vi "0716206_calculator_without_formula.vi"() -> ()   [LabVIEW 2021]
uses:
  <vilib>/Utility/miscctls.llb/LVDateTimeRec.ctl
panel:
  out "date time rec":T1
  out "stack":dbl[](array[numeric])
  out "is_neg":bool=TRUE
  out "Array operator":string[](array[string])
  out "buffer":string
  out "Array number":dbl[](array[numeric])
  out "Power":bool
  out "Storage2 ans":dbl format="%#_13g"
  out "Storage1 ans":dbl format="%#_13g"
  out "B":bool=TRUE
  out "Storage2":string
  out "Storage1":string
  out "Error":string
  out "Ans":dbl format="%#_13g"
  out "System Time":string
  out "Execution Time (s)":dbl caption="Elapsed Time (s)"
  out "String":string
  in  "Cluster":T2
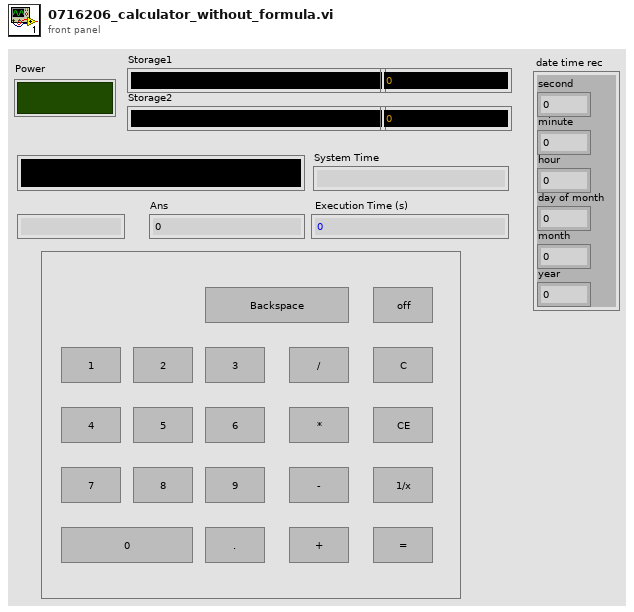
[diagram p1: front panel]
types:
  T1 = typedef "LVDateTimeRec.ctl" = cluster{"fractional second":dbl, "second":i32, "minute":i32, "hour":i32, "day of month":i32, "month":i32, "year":i32, "day of week":i32, "day of year":i32, "DST":i32}
  T2 = cluster{bool, bool, bool, bool, bool, bool, bool, bool, bool, bool, bool, bool, bool, bool, bool, bool, bool, bool, bool, bool, bool, bool, bool, bool}
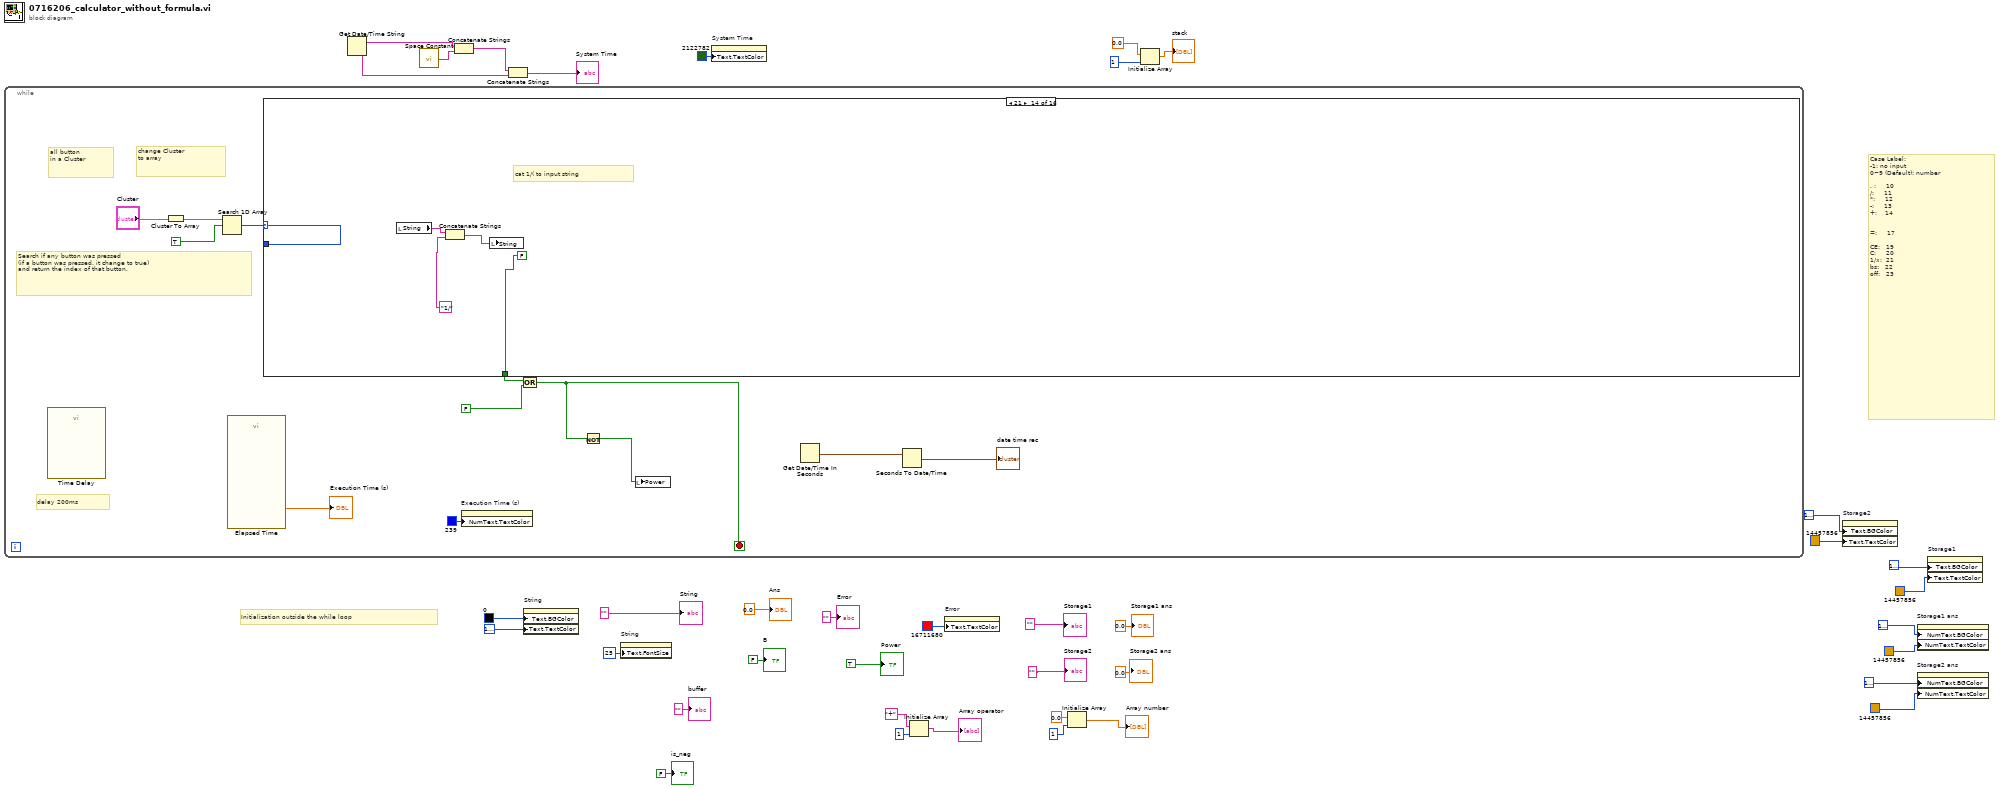
[diagram p0: block diagram]
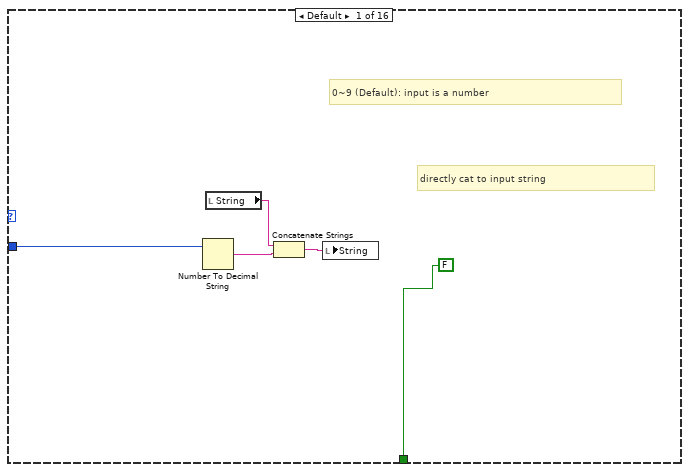
[diagram p2: hidden frame]
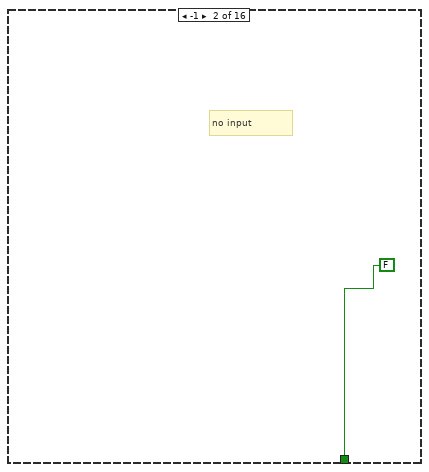
[diagram p3: hidden frame]
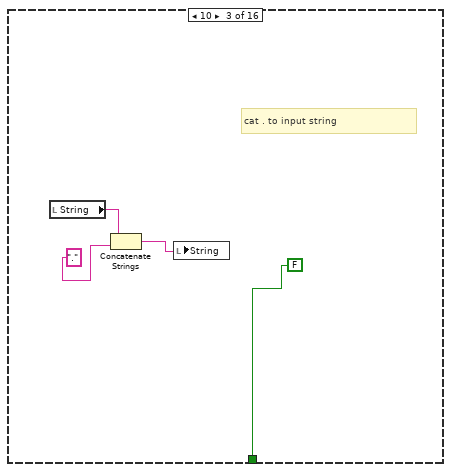
[diagram p4: hidden frame]
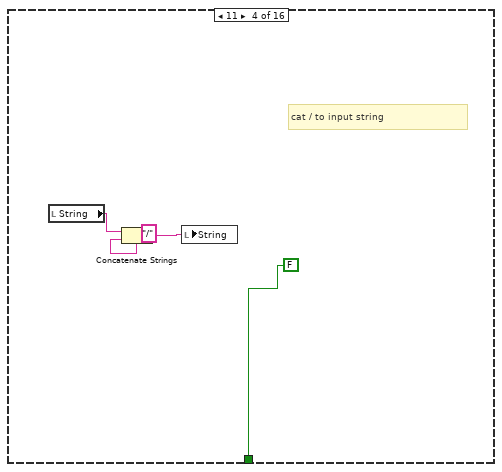
[diagram p5: hidden frame]
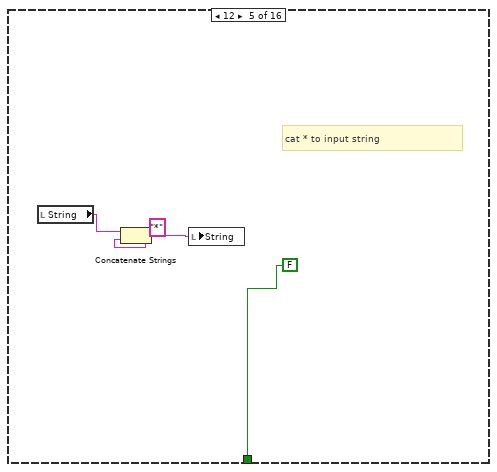
[diagram p6: hidden frame]
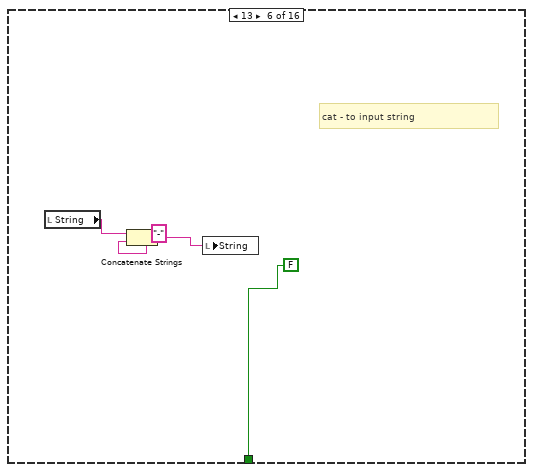
[diagram p7: hidden frame]
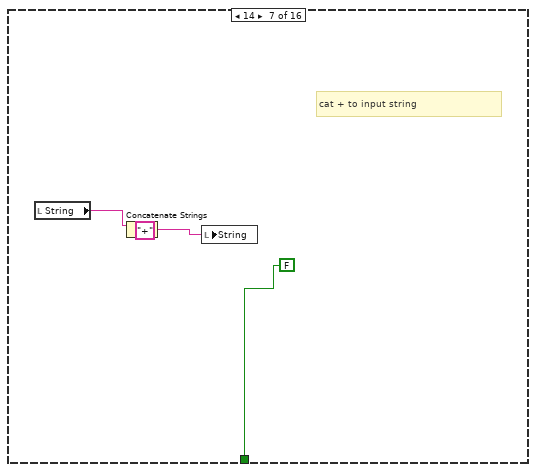
[diagram p8: hidden frame]
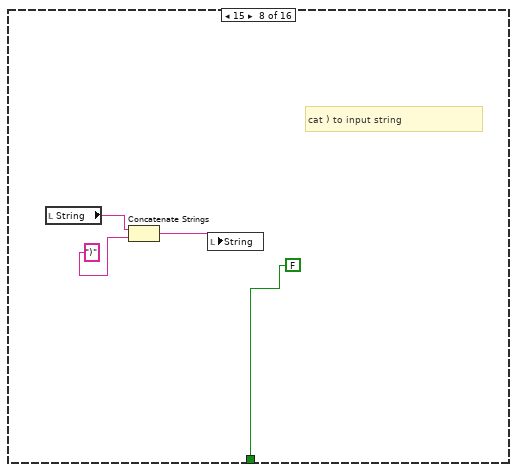
[diagram p9: hidden frame]
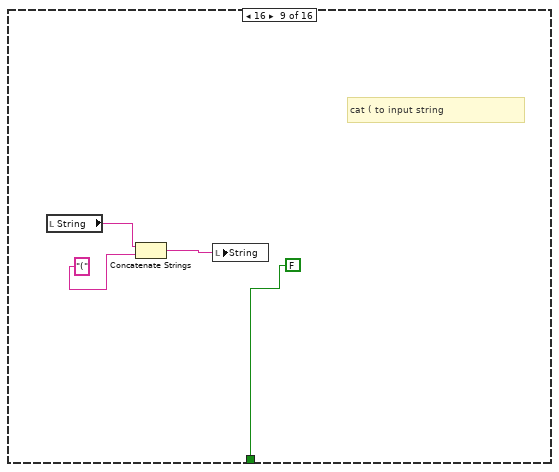
[diagram p10: hidden frame]
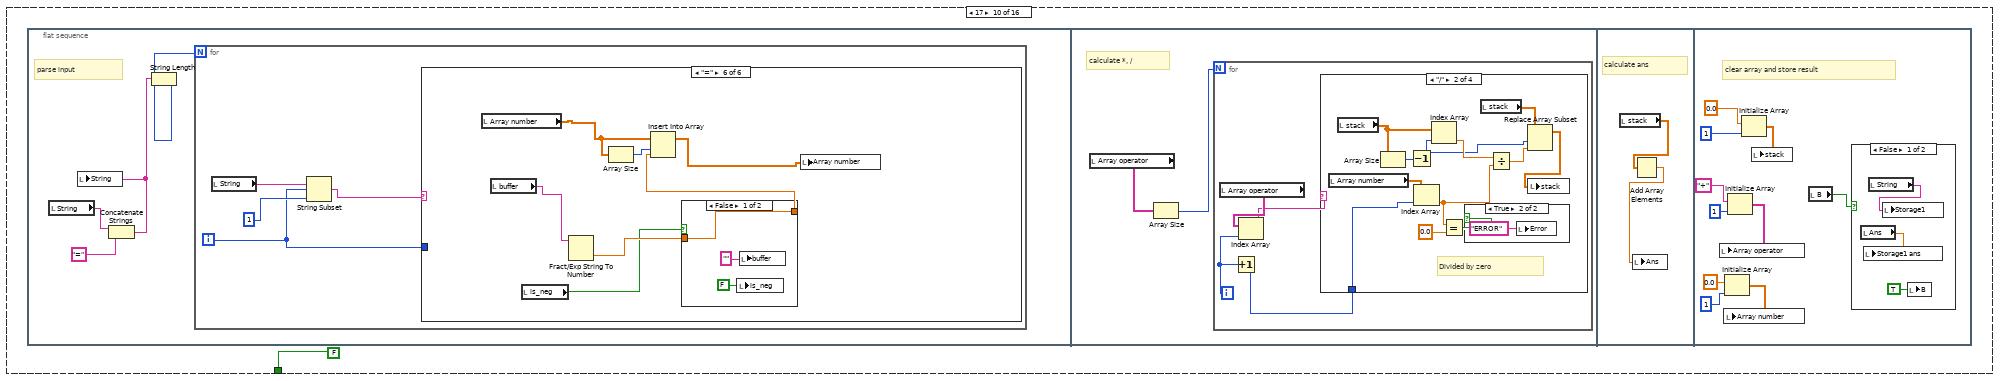
[diagram p11: hidden frame]
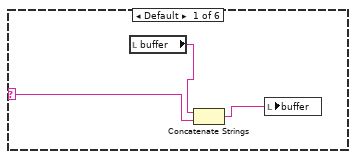
[diagram p12: hidden frame]
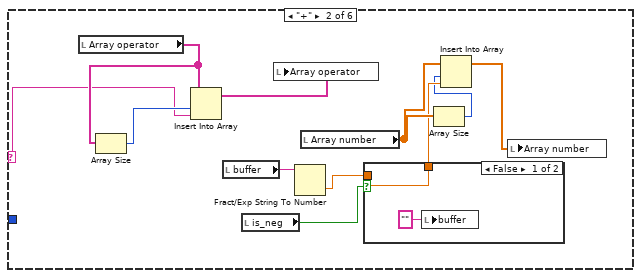
[diagram p13: hidden frame]
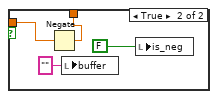
[diagram p14: hidden frame]
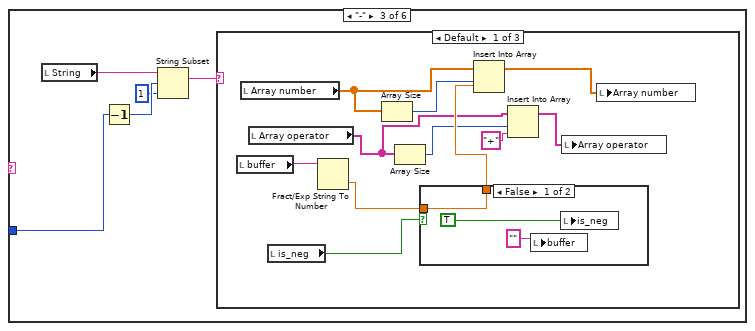
[diagram p15: hidden frame]
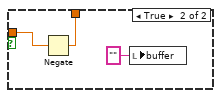
[diagram p16: hidden frame]
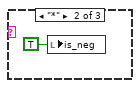
[diagram p17: hidden frame]
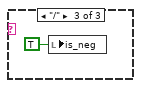
[diagram p18: hidden frame]
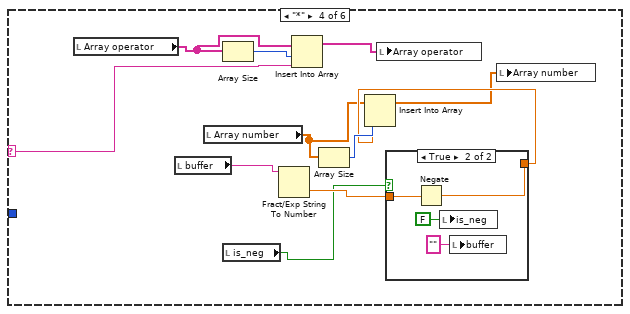
[diagram p19: hidden frame]
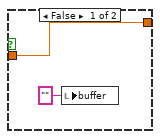
[diagram p20: hidden frame]
diagram:
  # "Initialization outside the while loop"
  # "Case Label:\n-1: no input\n0~9 (Default): number\n\n. :     10\n/:     11\n*:     12\n-:     13\n+:    14\n \n \n=:     17\n\nCE:   19\nC:     20\n1/x:  21\nbs:   22\noff:   23"
  n1 = while {
    stop <- w41 stop-if-true
    # "Search if any button was pressed\n(if a button was pressed, it change to true)\nand return the index of that button."
    # "change Cluster \nto array"
    # "all button \nin a Cluster"
    # "delay 200ms"
    n2 = call "Time Delay"() -> ()  [unwired: 11 in, 1 out]
    n3 = Cluster To Array(cluster="Cluster") -> (array=w49:bool[])
    n4 = Search 1D Array(1D array=w49, element=TRUE) -> (index of element=w47:i32)  [unwired: 1 in]
    n5 = call "Elapsed Time"() -> ("Elapsed Time (s)"=→"Execution Time (s)":dbl)  [unwired: 12 in, 7 out]
    n6 = case shown="21" w47 {
      tunnel: w47 -> [w52 _ _ _ _ _ _ _ _ _ _ _ _ _ _ _]
      tunnel: [FALSE FALSE FALSE FALSE FALSE FALSE FALSE FALSE FALSE FALSE FALSE FALSE FALSE FALSE FALSE TRUE] -> w46
      frame Default {
        # "directly cat to input string"
        # "0~9 (Default): input is a number"
        n7 = Number To Decimal String(number=w52) -> (decimal integer string=w53:string)  [unwired: 1 in]
        n8 = local read "String"() -> (w54:string)
        n9 = Concatenate Strings(w54, w53) -> (w55:string)
        n10 = local write "String"(w55) -> ()
      }
      frame -1 {
        # "no input"
      }
      frame 10 {
        # "cat . to input string"
        n11 = local read "String"() -> (w60:string)
        n12 = Concatenate Strings(w60, "." ("string")) -> (w59:string)
        n13 = local write "String"(w59) -> ()
      }
      frame 11 {
        # "cat / to input string"
        n14 = local read "String"() -> (w64:string)
        n15 = Concatenate Strings(w64, "/" ("string")) -> (w62:string)
        n16 = local write "String"(w62) -> ()
      }
      frame 12 {
        # "cat * to input string"
        n17 = local read "String"() -> (w68:string)
        n18 = Concatenate Strings(w68, "*" ("string")) -> (w66:string)
        n19 = local write "String"(w66) -> ()
      }
      frame 13 {
        # "cat - to input string"
        n20 = local read "String"() -> (w72:string)
        n21 = Concatenate Strings(w72, "-" ("string")) -> (w70:string)
        n22 = local write "String"(w70) -> ()
      }
      frame 14 {
        # "cat + to input string"
        n23 = local read "String"() -> (w76:string)
        n24 = Concatenate Strings(w76, "+" ("string")) -> (w75:string)
        n25 = local write "String"(w75) -> ()
      }
      frame 15 {
        # "cat ) to input string"
        n26 = local read "String"() -> (w79:string)
        n27 = Concatenate Strings(w79, ")" ("string")) -> (w80:string)
        n28 = local write "String"(w80) -> ()
      }
      frame 16 {
        # "cat ( to input string"
        n29 = local read "String"() -> (w83:string)
        n30 = Concatenate Strings(w83, "(" ("string")) -> (w84:string)
        n31 = local write "String"(w84) -> ()
      }
      frame 17 {
        n32 = flat-sequence {
          frame #0 {
            # "parse input"
            n33 = local read "String"() -> (w88:string)
            n34 = Concatenate Strings(w88, "=" ("string")) -> (w89:string)
            n35 = local write "String"(w89) -> ()
            n36 = String Length(string=w89) -> (length=w87:i32)
            n37 = for {
              N: w87 -> [_]
              i -> [w90]
              n38 = local read "String"() -> (w92:string)
              n39 = String Subset(string=w92, offset (0)=w90, length (rest)=1 ("length (rest)")) -> (substring=w91:string)
              n40 = case shown="\"=\"" w91 {
                selector: w91 -> [w94 w104 _ w147 w164 _]
                tunnel: w90 -> [_ _ w118 _ _ _]
                frame Default {
                  n41 = local read "buffer"() -> (w95:string)
                  n42 = Concatenate Strings(w95, w94) -> (w96:string)
                  n43 = local write "buffer"(w96) -> ()
                }
                frame "+" {
                  n44 = local read "Array operator"() -> (w107:string[])
                  n45 = Array Size(array=w107) -> (size(s)=w106:i32)
                  n46 = Insert Into Array(array=w107, index=w106, new element=w104) -> (w105:string[])
                  n47 = local read "buffer"() -> (w103:string)
                  n48 = local read "is_neg"() -> (w102:bool)
                  n49 = local write "Array operator"(w105) -> ()
                  n50 = Fract/Exp String To Number(string=w103) -> (number=w101:dbl)  [unwired: 3 in, 1 out]
                  n51 = local read "Array number"() -> (w100:dbl[])
                  n52 = case shown="False" w102 {
                    tunnel: w101 -> [w109 w113]
                    tunnel: [w109 w112] -> w99
                    frame False {
                      n53 = local write "buffer"("" ("buffer")) -> ()
                    }
                    frame True {
                      n54 = Negate(x=w113) -> (-x=w112:dbl)
                      n55 = local write "buffer"("" ("buffer")) -> ()
                      n56 = local write "is_neg"(FALSE ("is_neg")) -> ()
                    }
                  }
                  n57 = Array Size(array=w100) -> (size(s)=w98:i32)
                  n58 = Insert Into Array(array=w100, index=w98, new element=w99) -> (w97:dbl[])
                  n59 = local write "Array number"(w97) -> ()
                }
                frame "-" {
                  n60 = local read "String"() -> (w115:string)
                  n61 = Decrement(x=w118) -> (x-1=w117:i32)
                  n62 = String Subset(string=w115, offset (0)=w117, length (rest)=1 ("length (rest)")) -> (substring=w114:string)
                  n63 = case shown="Default" w114 {
                    frame Default {
                      n64 = local read "buffer"() -> (w125:string)
                      n65 = local read "Array number"() -> (w124:dbl[])
                      n66 = local read "Array operator"() -> (w120:string[])
                      n67 = local read "is_neg"() -> (w126:bool)
                      n68 = Fract/Exp String To Number(string=w125) -> (number=w127:dbl)  [unwired: 3 in, 1 out]
                      n69 = Array Size(array=w124) -> (size(s)=w128:i32)
                      n70 = Array Size(array=w120) -> (size(s)=w122:i32)
                      n71 = case shown="False" w126 {
                        tunnel: w127 -> [w132 w135]
                        tunnel: [w132 w134] -> w129
                        frame False {
                          n72 = local write "buffer"("" ("buffer")) -> ()
                          n73 = local write "is_neg"(TRUE ("is_neg")) -> ()
                        }
                        frame True {
                          n74 = Negate(x=w135) -> (-x=w134:dbl)
                          n75 = local write "buffer"("" ("buffer")) -> ()
                        }
                      }
                      n76 = Insert Into Array(array=w124, index=w128, new element=w129) -> (w123:dbl[])
                      n77 = Insert Into Array(array=w120, index=w122, new element="+") -> (w119:string[])
                      n78 = local write "Array operator"(w119) -> ()
                      n79 = local write "Array number"(w123) -> ()
                    }
                    frame "*" {
                      n80 = local write "is_neg"(TRUE ("is_neg")) -> ()
                    }
                    frame "/" {
                      n81 = local write "is_neg"(TRUE ("is_neg")) -> ()
                    }
                  }
                }
                frame "*" {
                  n82 = local read "Array operator"() -> (w145:string[])
                  n83 = local read "buffer"() -> (w141:string)
                  n84 = local read "Array number"() -> (w139:dbl[])
                  n85 = Array Size(array=w145) -> (size(s)=w148:i32)
                  n86 = local read "is_neg"() -> (w140:bool)
                  n87 = Fract/Exp String To Number(string=w141) -> (number=w143:dbl)  [unwired: 3 in, 1 out]
                  n88 = Insert Into Array(array=w145, index=w148, new element=w147) -> (w146:string[])
                  n89 = Array Size(array=w139) -> (size(s)=w144:i32)
                  n90 = local write "Array operator"(w146) -> ()
                  n91 = case shown="True" w140 {
                    tunnel: w143 -> [w150 w154]
                    tunnel: [w150 w153] -> w142
                    frame False {
                      n92 = local write "buffer"("" ("buffer")) -> ()
                    }
                    frame True {
                      n93 = Negate(x=w154) -> (-x=w153:dbl)
                      n94 = local write "is_neg"(FALSE ("is_neg")) -> ()
                      n95 = local write "buffer"("" ("buffer")) -> ()
                    }
                  }
                  n96 = Insert Into Array(array=w139, index=w144, new element=w142) -> (w138:dbl[])
                  n97 = local write "Array number"(w138) -> ()
                }
                frame "/" {
                  n98 = local read "Array operator"() -> (w163:string[])
                  n99 = local read "buffer"() -> (w157:string)
                  n100 = local read "Array number"() -> (w156:dbl[])
                  n101 = Array Size(array=w163) -> (size(s)=w165:i32)
                  n102 = Fract/Exp String To Number(string=w157) -> (number=w160:dbl)  [unwired: 3 in, 1 out]
                  n103 = local read "is_neg"() -> (w158:bool)
                  n104 = Array Size(array=w156) -> (size(s)=w161:i32)
                  n105 = Insert Into Array(array=w163, index=w165, new element=w164) -> (w162:string[])
                  n106 = local write "Array operator"(w162) -> ()
                  n107 = case shown="False" w158 {
                    tunnel: w160 -> [w167 w171]
                    tunnel: [w167 w170] -> w159
                    frame False {
                      n108 = local write "buffer"("" ("buffer")) -> ()
                    }
                    frame True {
                      n109 = Negate(x=w171) -> (-x=w170:dbl)
                      n110 = local write "is_neg"(FALSE ("is_neg")) -> ()
                      n111 = local write "buffer"("" ("buffer")) -> ()
                    }
                  }
                  n112 = Insert Into Array(array=w156, index=w161, new element=w159) -> (w155:dbl[])
                  n113 = local write "Array number"(w155) -> ()
                }
                frame "=" {
                  n114 = local read "Array number"() -> (w173:dbl[])
                  n115 = local read "buffer"() -> (w175:string)
                  n116 = local read "is_neg"() -> (w174:bool)
                  n117 = Fract/Exp String To Number(string=w175) -> (number=w177:dbl)  [unwired: 3 in, 1 out]
                  n118 = Array Size(array=w173) -> (size(s)=w178:i32)
                  n119 = case shown="False" w174 {
                    tunnel: w177 -> [w181 w185]
                    tunnel: [w181 w184] -> w176
                    frame False {
                      n120 = local write "is_neg"(FALSE ("is_neg")) -> ()
                      n121 = local write "buffer"("" ("buffer")) -> ()
                    }
                    frame True {
                      n122 = Negate(x=w185) -> (-x=w184:dbl)
                      n123 = local write "buffer"("" ("buffer")) -> ()
                      n124 = local write "is_neg"(FALSE ("is_neg")) -> ()
                    }
                  }
                  n125 = Insert Into Array(array=w173, index=w178, new element=w176) -> (w172:dbl[])
                  n126 = local write "Array number"(w172) -> ()
                }
              }
            }
          }
          frame #1 {
            # "calculate *, /"
            n127 = local read "Array operator"() -> (w187:string[])
            n128 = Array Size(array=w187) -> (size(s)=w186:i32)
            n129 = for {
              N: w186 -> [_]
              i -> [w188]
              n130 = local read "Array operator"() -> (w191:string[])
              n131 = Increment(x=w188) -> (x+1=w189:i32)
              n132 = Index Array(array=w191, index=w188) -> (element=w190:string)
              n133 = case shown="\"/\"" w190 {
                tunnel: w189 -> [w200 w210 _ w220]
                frame "*" {
                  n134 = local read "stack"() -> (w198:dbl[])
                  n135 = local read "Array number"() -> (w201:dbl[])
                  n136 = Index Array(array=w201, index=w200) -> (element=w196:dbl)
                  n137 = Array Size(array=w198) -> (size(s)=w199:i32)
                  n138 = Decrement(x=w199) -> (x-1=w194:i32)
                  n139 = Index Array(array=w198, index=w194) -> (element=w197:dbl)
                  n140 = Multiply(x=w197, y=w196) -> (x*y=w195:dbl)
                  n141 = local read "stack"() -> (w192:dbl[])
                  n142 = Replace Array Subset(array=w192, new element=w195, index=w194) -> (w193:dbl[])
                  n143 = local write "stack"(w193) -> ()
                }
                frame "/" {
                  # "Divided by zero"
                  n144 = local read "Array number"() -> (w209:dbl[])
                  n145 = local read "stack"() -> (w211:dbl[])
                  n146 = Array Size(array=w211) -> (size(s)=w212:i32)
                  n147 = Decrement(x=w212) -> (x-1=w207:i32)
                  n148 = Index Array(array=w209, index=w210) -> (element=w203:dbl)
                  n149 = Index Array(array=w211, index=w207) -> (element=w213:dbl)
                  n150 = Equal?(x=w203, y=0.0) -> (x = y?=w202:bool)
                  n151 = case shown="True" w202 {
                    frame False {
                    }
                    frame True {
                      n152 = local write "Error"("ERROR" ("Error")) -> ()
                    }
                  }
                  n153 = local read "stack"() -> (w206:dbl[])
                  n154 = Divide(x=w213, y=w203) -> (x/y=w208:dbl)
                  n155 = Replace Array Subset(array=w206, new element=w208, index=w207) -> (w205:dbl[])
                  n156 = local write "stack"(w205) -> ()
                }
                frame Default {
                }
                frame "+" {
                  n157 = local read "Array number"() -> (w219:dbl[])
                  n158 = local read "stack"() -> (w216:dbl[])
                  n159 = Array Size(array=w216) -> (size(s)=w218:i32)
                  n160 = Index Array(array=w219, index=w220) -> (element=w217:dbl)
                  n161 = Insert Into Array(array=w216, index=w218, new element=w217) -> (w215:dbl[])
                  n162 = local write "stack"(w215) -> ()
                }
              }
            }
          }
          frame #2 {
            # "calculate ans"
            n163 = local read "stack"() -> (w222:dbl[])
            n164 = Add Array Elements(numeric array=w222) -> (sum=w221:dbl)
            n165 = local write "Ans"(w221) -> ()
          }
          frame #3 {
            # "clear array and store result"
            n166 = Initialize Array(0.0 ("element"), 1 ("dimension size")) -> (w224:dbl[])
            n167 = local write "Array number"(w224) -> ()
            n168 = Initialize Array("+", 1 ("dimension size")) -> (w227:string[])
            n169 = local write "Array operator"(w227) -> ()
            n170 = Initialize Array(0.0 ("element"), 1 ("dimension size")) -> (w230:dbl[])
            n171 = local write "stack"(w230) -> ()
            n172 = local read "B"() -> (w223:bool)
            n173 = case shown="False" w223 {
              frame False {
                n174 = local read "Ans"() -> (w233:dbl)
                n175 = local write "Storage1 ans"(w233) -> ()
                n176 = local read "String"() -> (w234:string)
                n177 = local write "Storage1"(w234) -> ()
                n178 = local write "B"(TRUE ("B")) -> ()
              }
              frame True {
                n179 = local read "Ans"() -> (w236:dbl)
                n180 = local write "Storage2 ans"(w236) -> ()
                n181 = local read "String"() -> (w237:string)
                n182 = local write "Storage2"(w237) -> ()
                n183 = local write "B"(FALSE ("B")) -> ()
              }
            }
          }
        }
      }
      frame 18 {
        # "cat sqrt( to input string"
        n184 = local read "String"() -> (w241:string)
        n185 = Concatenate Strings(w241, "sqrt(" ("string")) -> (w242:string)
        n186 = local write "String"(w242) -> ()
      }
      frame 19 {
        # "clear error message, ans"
        n187 = local write "Error"("" ("Error")) -> ()
        n188 = local write "Ans"(0.0 ("Ans")) -> ()
        n189 = Initialize Array(0.0 ("element"), 1 ("dimension size")) -> (w243:dbl[])
        n190 = Initialize Array("+", 1 ("dimension size")) -> (w246:string[])
        n191 = local write "Array number"(w243) -> ()
        n192 = local write "Array operator"(w246) -> ()
      }
      frame 20 {
        w258 = "" ("String")
        # "clear error message, ans, input"
        n193 = local write "Ans"(0.0 ("Ans")) -> ()
        n194 = local write "String"(w258) -> ()
        n195 = local write "Error"(w258) -> ()
        n196 = Initialize Array(0.0 ("element"), 1 ("dimension size")) -> (w252:dbl[])
        n197 = Initialize Array("+", 1 ("dimension size")) -> (w255:string[])
        n198 = local write "Array number"(w252) -> ()
        n199 = local write "Array operator"(w255) -> ()
      }
      frame 21 {
        # "cat 1/( to input string"
        n200 = local read "String"() -> (w263:string)
        n201 = Concatenate Strings(w263, "1/" ("string")) -> (w264:string)
        n202 = local write "String"(w264) -> ()
      }
      frame 22 {
        # "pop back a char in input string using string replace: replace the last char by an empty\nstring of length 1"
        n203 = local read "String"() -> (w266:string)
        n204 = String Length(string=w266) -> (length=w269:i32)
        n205 = Decrement(x=w269) -> (x-1=w270:i32)
        n206 = Replace Substring(2:1 ("length (len. of substring)"), 3:w270, 4:"" ("substring (\"\")"), 5:w266) -> (1:w271:string)  [unwired: 1 out]
        n207 = local write "String"(w271) -> ()
      }
      frame 23 {
        # "turn the calc off: break the loop"
      }
    }
    n208 = property on="Execution Time (s)" class="DigNum (strict)"("NumText.TextColor"=u32 239 ("Numeric Text.Text Colors:Text Color")) -> ()  [unwired: 2 in, 2 out]
    n209 = Or(x=w46, y=FALSE) -> (x .or. y?=w41:bool)
    n210 = Not(x=w41) -> (.not. x?=w42:bool)
    n211 = local write "Power"(w42) -> ()
    n212 = Get Date/Time In Seconds() -> (seconds since 1Jan1904=w39:timestamp)
    n213 = Seconds To Date/Time(time stamp (now)=w39) -> (date time rec=→"date time rec":T1)  [unwired: 1 in]
  }
  n214 = Get Date/Time String() -> (date string=w36:string, time string=w34:string)  [unwired: 3 in]
  n215 = call <vilib>:"Space Constant.vi"() -> ("String"=w37:string)
  n216 = Concatenate Strings(w36, w37) -> (w35:string)
  n217 = Concatenate Strings(w35, w34) -> (→"System Time":string)
  n218 = property on="String" class="Str"("Text.BGColor"=u32 0 ("Text.Text Colors:BG Color"), "Text.TextColor"=u32 16777238 ("Text.Text Colors:Text Color")) -> ()  [unwired: 2 in, 2 out]
  n219 = property on="String" class="Str"("Text.FontSize"=u32 25 ("Text.Font:Size")) -> ()  [unwired: 2 in, 2 out]
  n220 = property on="System Time" class="Str"("Text.TextColor"=u32 2122782 ("Text.Text Colors:Text Color")) -> ()  [unwired: 2 in, 2 out]
  n221 = Initialize Array("+", 1 ("dimension size")) -> (→"Array operator":string[])
  n222 = property on="Error" class="Str"("Text.TextColor"=u32 16711680 ("Text.Text Colors:Text Color")) -> ()  [unwired: 2 in, 2 out]
  n223 = Initialize Array(0.0 ("element"), 1 ("dimension size")) -> (→"Array number":dbl[])
  n224 = Initialize Array(0.0 ("element"), 1 ("dimension size")) -> (→"stack":dbl[])
  n225 = property on="Storage2" class="Str"("Text.BGColor"=u32 16777222 ("Text.Text Colors:BG Color"), "Text.TextColor"=u32 14457856 ("Text.Text Colors:Text Color")) -> ()  [unwired: 2 in, 2 out]
  n226 = property on="Storage1 ans" class="DigNum (strict)"("NumText.BGColor"=u32 16777222 ("Text.Text Colors:BG Color"), "NumText.TextColor"=u32 14457856 ("Text.Text Colors:Text Color")) -> ()  [unwired: 2 in, 2 out]
  n227 = property on="Storage2 ans" class="DigNum (strict)"("NumText.BGColor"=u32 16777222 ("Text.Text Colors:BG Color"), "NumText.TextColor"=u32 14457856 ("Text.Text Colors:Text Color")) -> ()  [unwired: 2 in, 2 out]
  n228 = property on="Storage1" class="Str"("Text.BGColor"=u32 16777222 ("Text.Text Colors:BG Color"), "Text.TextColor"=u32 14457856 ("Text.Text Colors:Text Color")) -> ()  [unwired: 2 in, 2 out]
  "String" <- ""
  "Ans" <- 0.0 ("Ans")
  "Error" <- "" ("Error")
  "Storage1" <- ""
  "Storage2" <- ""
  "B" <- FALSE ("Boolean")
  "Storage1 ans" <- 0.0 ("Storage1 ans")
  "Storage2 ans" <- 0.0 ("Storage2 ans")
  "Power" <- TRUE ("Power")
  "buffer" <- ""
  "is_neg" <- FALSE ("is_neg")
